vi "Get Properties.vi"(8 "error in":errorcluster, 11 "VI Name":string caption="VI Name (\"\")") -> (0 "error out":errorcluster, 1 "Column Data Type":enum16{"String", "Numeric"}[](array[ring]), 2 "Column Labels":string[](array[string])=["VI Name", "State", "Reentrant", "Reentrancy Type", "FP Behavior", "Code Size", "Data Size", "VI Path"], 3 "VI Name Out":string, 4 "VI Properties":string[](array[string]))   [LabVIEW 2013]
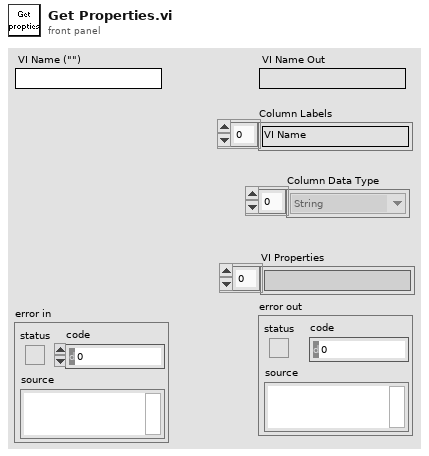
[diagram p1: front panel]
types:
  T1 = enum32{"Bad", "Idle", "Run top level", "Running"}
  T2 = enum16{"Share clones between instances", "Preallocate clone for each instance"}
  T3 = enum32{"Invalid", "Default", "Floating", "Floating/Auto-Hide", "Modal"}
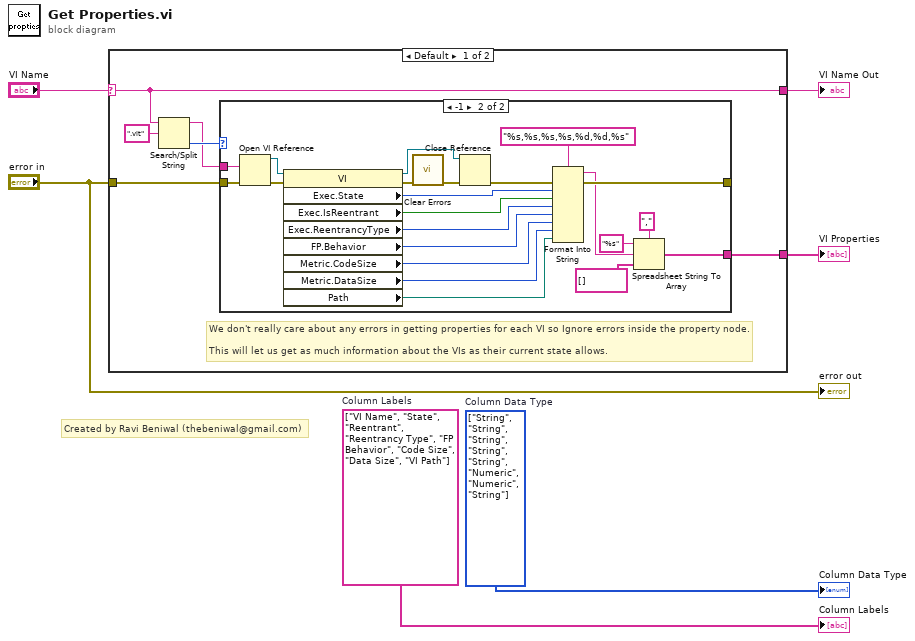
[diagram p0: block diagram]
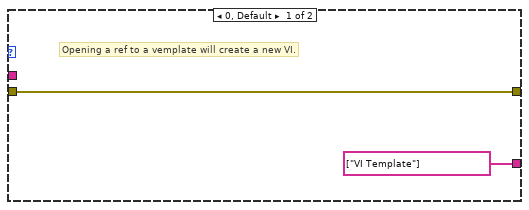
[diagram p2: hidden frame]
diagram:
  w1 = enum16{"String", "Numeric"}[] [enum."String", enum."String", enum."String", enum."String", enum."String", enum."Numeric", enum."Numeric", enum."String"] items=["String", "Numeric"]  # Column Data Type
  w5 = string[] ["VI Name", "State", "Reentrant", "Reentrancy Type", "FP Behavior", "Code Size", "Data Size", "VI Path"]  # Column Labels
  # "Created by Ravi Beniwal (thebeniwal@gmail.com)"
  n1 = case shown="Default" "VI Name" {
    selector: "VI Name" -> [w7 w37]
    tunnel: [w12 _] -> w6
    tunnel: "error in" -> [w8 _]
    tunnel: [w7 w37] -> w3
    frame Default {
      # "We don't really care about any errors in getting properties for each VI so Ignore errors inside the property node.\n\nThis will let us get as much information about the VIs as their current state allows."
      n2 = Search/Split String(string=w7, search string/char (-)=".vit") -> (substring before match=w10:string, offset of match=w11:i32)  [unwired: 2 out]
      n3 = case shown="-1" w11 {
        tunnel: w8 -> [w14 w34]
        tunnel: [w14 w22] -> _
        tunnel: w10 -> [_ w31]
        tunnel: [string[] ["VI Template"] w27] -> w12
        frame 0, Default {
          # "Opening a ref to a vemplate will create a new VI."
        }
        frame -1 {
          n4 = Open VI Reference(vi path=w31, error in (no error)=w34) -> (vi reference=w36:refnum<vi>, error out=w35:errorcluster)  [unwired: 4 out]
          n5 = property class="VI"(reference=w36, error in=w35) -> (reference out=w33:refnum<vi>, error out=w32:errorcluster, "Exec.State"=w30:T1, "Exec.IsReentrant"=w29:bool, "Exec.ReentrancyType"=w25:T2, "FP.Behavior"=w24:T3, "Metric.CodeSize"=w21:u32, "Metric.DataSize"=w20:u32, "Path"=w19:path)
          n6 = call <vilib>:"Clear Errors.vi"("error in (no error)"=w32) -> ("error out"=w15:errorcluster)  [unwired: 6 in]
          n7 = Close Reference(reference=w33, error in (no error)=w15) -> (error out=w23:errorcluster)
          n8 = Format Into String(format string="%s,%s,%s,%s,%d,%d,%s", error in=w23, w30, w29, w25, w24, w21, w20, w19) -> (resulting string=w16:string, error out=w22:errorcluster)  [unwired: 1 in]
          n9 = Spreadsheet String To Array(delimiter (Tab)=",", format string="%s", spreadsheet string=w16, array type (2D Dbl)=string[] [] ("appended array")) -> (array=w27:string[])
        }
      }
    }
    frame "" {
      # "Addin this blank case let's us use this VI for getting the Col headers. \nIt is just easier to manage the column headers and getting their values in one VI."
    }
  }
  "VI Properties" <- w6
  "VI Name Out" <- w3
  "error out" <- "error in"
  "Column Labels" <- w5
  "Column Data Type" <- w1
